vi "ASIC_CONFIGURAR add MUX.vi"(7 "Espera acceso USB":u32=10, 8 "error in":errorcluster, 9 "BUFF_ENA":bool, 10 "ADD mux(0..3)":T1, 11 "ftHandle_in":u32) -> (0 "error out":errorcluster, 3 "ftHandle_out":u32)   [LabVIEW 2019]
uses:
  ASIC_Valores ADD_MUX_ena.ctl
panel:
  out "test":u16 format="%04x"
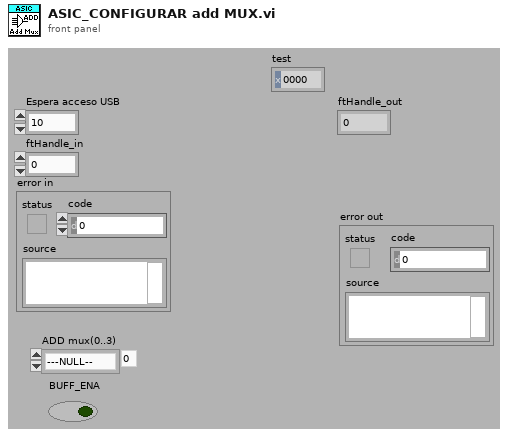
[diagram p1: front panel]
types:
  T1 = typedef "ASIC_Valores ADD_MUX_ena.ctl" = enum16{"---NULL--", "ADD A", "ADD B", "ADD C"}
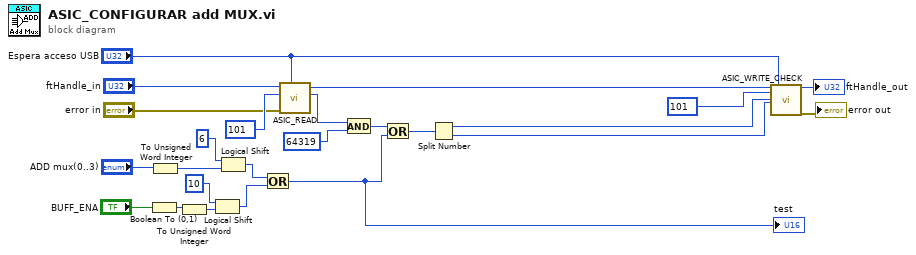
[diagram p0: block diagram]
diagram:
  n1 = Boolean To (0,1)(Boolean="BUFF_ENA") -> (0, 1=w5:i16)
  n2 = To Unsigned Word Integer(number="ADD mux(0..3)") -> (unsigned 16bit integer=w8:u16)
  n3 = To Unsigned Word Integer(number=w5) -> (unsigned 16bit integer=w6:u16)
  n4 = Logical Shift(y=u16 10 ("x"), x=w6) -> (x << y=w2:u16)
  n5 = Logical Shift(y=u16 6 ("x"), x=w8) -> (x << y=w3:u16)
  n6 = Or(x=w3, y=w2) -> (x .or. y?=w1:u16)
  "test" <- w1
  n7 = call "ASIC_READ.vi"("Espera acceso USB"="Espera acceso USB", "error in"="error in", "Direccion Registro Asic"=u8 101, "ftHandle_in"="ftHandle_in") -> ("Valor Asic"=w13:u16, "ftHandle_out"=w16:u32)  [unwired: 5 in, 1 out]
  n8 = And(x=w13, y=u16 64319) -> (x .and. y?=w11:u16)
  n9 = Or(x=w11, y=w1) -> (x .or. y?=w10:u16)
  n10 = Split Number(x=w10) -> (hi(x)=w15:u8, lo(x)=w14:u8)
  n11 = call "ASIC_WRITE_CHECK.vi"("ftHandle_in"=w16, "Direccion Registro Asic"=u8 101, "Byte Alto"=w15, "Byte Bajo"=w14, "Espera acceso USB 2"="Espera acceso USB") -> ("ftHandle_out"=→"ftHandle_out":u32, "error out"=→"error out":errorcluster)  [unwired: 12 in, 1 out]
